vi "FTW-CodeGen-TraverseGObjects.vi"(0 "GObject to Traverse":refnum<vi>, 2 "GObject Filter Callback":refnum<vi>, 5 "Class Name":string, 7 "Initial Context":variant, 11 "error in":errorcluster) -> (8 "Final Context":variant, 15 "error out":errorcluster)   [LabVIEW 2015]
panel:
  # "Inputs"
  # "Outputs"
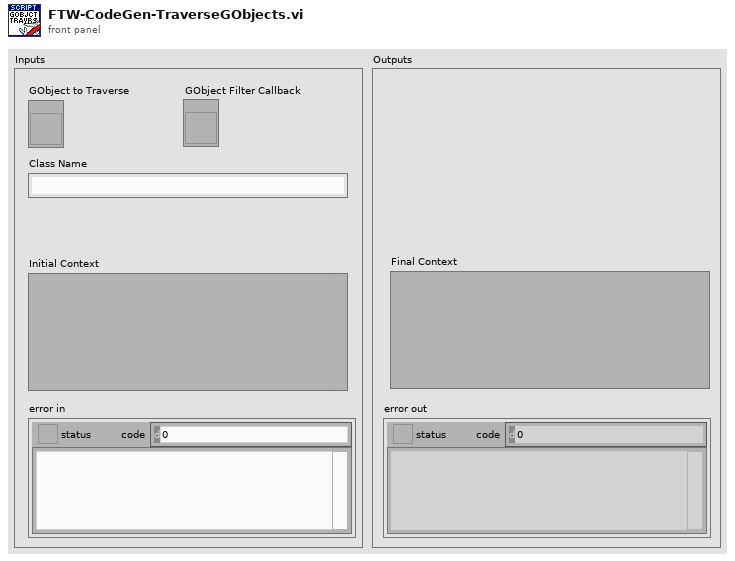
[diagram p1: front panel]
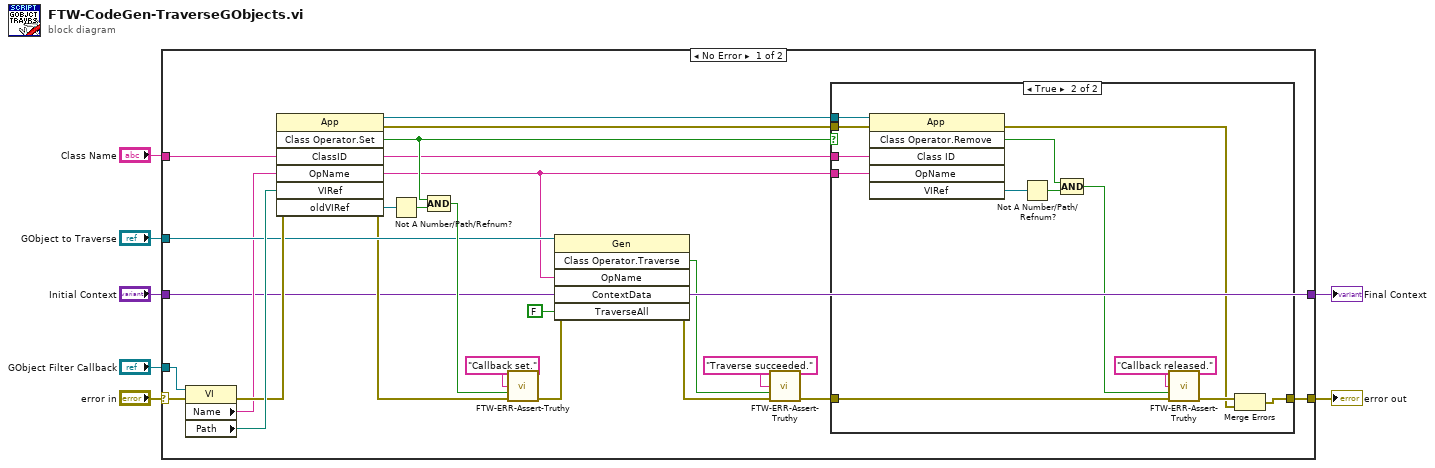
[diagram p0: block diagram]
diagram:
  n1 = case shown="No Error" "error in" {
    selector: "error in" -> [w28 w46]
    tunnel: "GObject to Traverse" -> [w23 _]
    tunnel: [w12 w45] -> w1
    tunnel: [w17 w46] -> w2
    tunnel: "Class Name" -> [w16 _]
    tunnel: "GObject Filter Callback" -> [w15 _]
    tunnel: "Initial Context" -> [w13 w45]
    frame No Error {
      n2 = property class="VI"(reference=w15, error in=w28) -> (error out=w29:errorcluster, "Name"=w14:string, "Path"=w30:path)  [unwired: 1 out]
      n3 = invoke class="App" method="Class Operator.Set"(error in=w29, "ClassID"=w16, "OpName"=w14, "VIRef"=w30) -> (reference out=w20:refnum<vi>, error out=w18:errorcluster, "SetClassOp"=w21:bool, "oldVIRef"=w26:refnum<vi>)  [unwired: 3 in, 3 out]
      n4 = Not A Number/Path/Refnum?(number/path/refnum=w26) -> (NaN/Path/Refnum?=w25:bool)
      n5 = Compound Arithmetic op=AND(w21, w25) -> (w24:bool)
      n6 = call "FTW-ERR-Assert-Truthy.vi"("Assertion"="Callback set.", "Assertion holds true?"=w24, "error in"=w18) -> ("error out"=w22:errorcluster)  [unwired: 12 in]
      n7 = invoke class="Gen" method="Class Operator.Traverse"(reference=w23, error in=w22, "OpName"=w14, "ContextData"=w13, "TraverseAll"=FALSE ("Traverse All")) -> (error out=w8:errorcluster, "Traverse"=w9:bool, "ContextData"=w12:variant)  [unwired: 1 in, 3 out]
      n8 = call "FTW-ERR-Assert-Truthy.vi"("Assertion"="Traverse succeeded.", "Assertion holds true?"=w9, "error in"=w8) -> ("error out"=w19:errorcluster)  [unwired: 12 in]
      n9 = case shown="True" w21 {
        tunnel: w20 -> [_ w43]
        tunnel: w16 -> [_ w42]
        tunnel: w14 -> [_ w41]
        tunnel: w19 -> [w31 w35]
        tunnel: w18 -> [_ w39]
        tunnel: [w31 w32] -> w17
        frame False {
        }
        frame True {
          n10 = invoke class="App" method="Class Operator.Remove"(reference=w43, error in=w39, "Class ID"=w42, "OpName"=w41) -> (error out=w33:errorcluster, "RemoveClassOp"=w38:bool, "VIRef"=w44:refnum<vi>)  [unwired: 2 in, 3 out]
          n11 = Not A Number/Path/Refnum?(number/path/refnum=w44) -> (NaN/Path/Refnum?=w37:bool)
          n12 = Compound Arithmetic op=AND(w38, w37) -> (w36:bool)
          n13 = call "FTW-ERR-Assert-Truthy.vi"("Assertion"="Callback released.", "Assertion holds true?"=w36, "error in"=w35) -> ("error out"=w34:errorcluster)  [unwired: 12 in]
          n14 = Merge Errors(w34, w33) -> (w32:errorcluster)
        }
      }
    }
    frame Error {
    }
  }
  "error out" <- w2
  "Final Context" <- w1
